vi "Temp Sensor.vi"() -> ()   [LabVIEW 2014]
uses:
  <vilib>/Utility/miscctls.llb/LVRectTypeDef.ctl
  Global Stop Program.vi
panel:
  out "Warning Ind.":bool
  in  "High Limit (°C)":dbl=70.0 format="%#_13g"
  out "Warning Txt":string
  in  "stop":bool
  out "Temperature (°C)":dbl
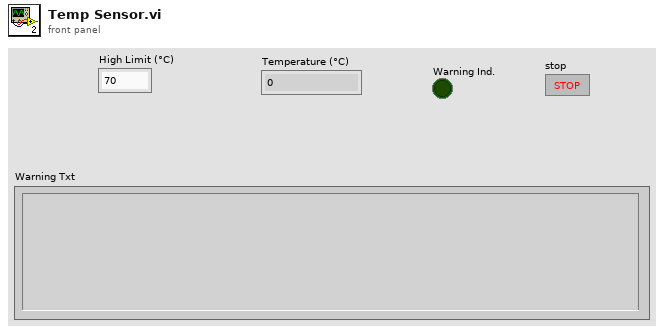
[diagram p1: front panel]
types:
  T1 = enum32{"Invalid", "Standard", "Closed", "Hidden", "Minimized", "Maximized"}
  T2 = typedef "LVRectTypeDef.ctl" = cluster{"Left":i16, "Top":i16, "Right":i16, "Bottom":i16}
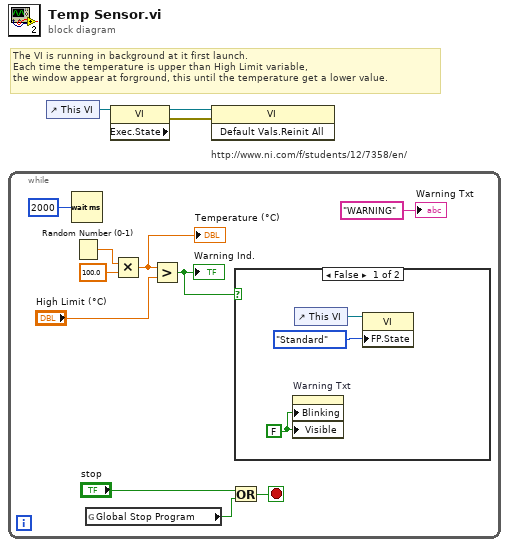
[diagram p0: block diagram]
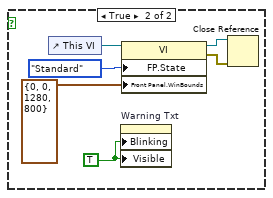
[diagram p2: hidden frame]
diagram:
  # "The VI is running in background at it first launch.\nEach time the temperature is upper than High Limit variable,\nthe window appear at forground, this until the temperature get a lower value."
  # "http://www.ni.com/f/students/12/7358/en/"
  n1 = while {
    stop <- w6 stop-if-true
    n2 = Wait (ms)(milliseconds to wait=u32 2000) -> ()  [unwired: 1 out]
    n3 = Random Number (0-1)() -> (number: 0 to 1=w13:dbl)
    n4 = global read "Global Stop Program.vi" "Global Stop Program"() -> (w4:bool)
    n5 = Multiply(x=w13, y=100.0) -> (x*y=w9:dbl)
    "Temperature (°C)" <- w9
    n6 = Greater?(x=w9, y="High Limit (°C)") -> (0:w8:bool)
    "Warning Ind." <- w8
    n7 = Or(x="stop", y=w4) -> (x .or. y?=w6:bool)
    n8 = case shown="False" w8 {
      frame False {
        w16 = FALSE
        n9 = property on="Warning Txt" class="Str"("Blinking"=w16, "Visible"=w16) -> ()  [unwired: 2 in, 2 out]
        n10 = control-ref of="This VI"() -> (w14:refnum<vi>)
        n11 = property class="VI"(reference=w14, "FP.State"=T1."Standard" ("Front Panel Window:State")) -> ()  [unwired: 1 in, 2 out]
      }
      frame True {
        w22 = TRUE
        n12 = control-ref of="This VI"() -> (w20:refnum<vi>)
        n13 = property on="Warning Txt" class="Str"("Blinking"=w22, "Visible"=w22) -> ()  [unwired: 2 in, 2 out]
        n14 = property class="VI"(reference=w20, "FP.State"=T1."Standard" ("Front Panel Window:State"), "Front Panel.WinBounds"=T2 {"Left"=0, "Top"=0, "Right"=1280, "Bottom"=800} ("Front Panel Window:Window Bounds")) -> (reference out=w17:refnum<vi>, error out=w18:errorcluster)  [unwired: 1 in]
        n15 = Close Reference(reference=w17, error in (no error)=w18) -> ()  [unwired: 1 out]
      }
    }
    "Warning Txt" <- "WARNING" ("Warning Txt")
  }
  n16 = control-ref of="This VI"() -> (w1:refnum<vi>)
  n17 = property class="VI" props=["Exec.State"](reference=w1) -> (reference out=w3:refnum<vi>, error out=w2:errorcluster)  [unwired: 1 in, 1 out]
  n18 = invoke class="VI" method="Default Vals.Reinit All"(reference=w3, error in=w2) -> ()  [unwired: 1 in, 3 out]
